vi "dvp Vi Refresh.vi"(11 "pCount":u32) -> (2 "function return":u32(ring), 3 "pCount out":u32)   [LabVIEW 2018, in "LabViewDVPCamera.lvlib"]
doc: "LabviewDvp2Api dvpStatus dvpViRefresh(dvpUint32 *pCount);"
uses:
  LabViewDVPCamera.lvlib
  LabViewDVPCamera/LabViewDVPCamera.dll
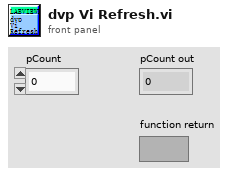
[diagram p1: front panel]
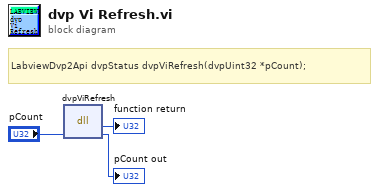
[diagram p0: block diagram]
diagram:
  # "LabviewDvp2Api dvpStatus dvpViRefresh(dvpUint32 *pCount);"
  n1 = dll-call lib="C:/Program Files (x86)/DVP2 Labview cn 64/Sample/LabViewDVPCamera/LabViewDVPCamera.*" fn="dvpViRefresh"("pCount"="pCount") -> (→"function return":u32, "pCount"=→"pCount out":u32)  [unwired: 3 in, 2 out]
